vi "Symphony Format Area.vi"(4 "Y Start":i32=255 min=1 max=255 step=1, 5 "Y End":i32=256 min=1 max=256 step=1, 6 "ImageMode":bool, 7 "error in (no error)":errorcluster, 8 "X Start":i32=1023 min=1 max=1023 step=1, 9 "X End":i32=1024 min=1 max=1024 step=1, 10 "numAreas":i32=1) -> (0 "error out":errorcluster, 2 "areas :":i32[][](array[numeric])=[[1], [1], [1], [1024], [256], [1], [256]], 3 "X Size Out":i32=1023 min=1 max=1023 step=1)   [LabVIEW 2019]
panel:
  # "Area#"
  # "X Origin"
  # "Y Origin"
  # "X Size"
  # "Y Size"
  # "X Bin"
  # "Y Bin"
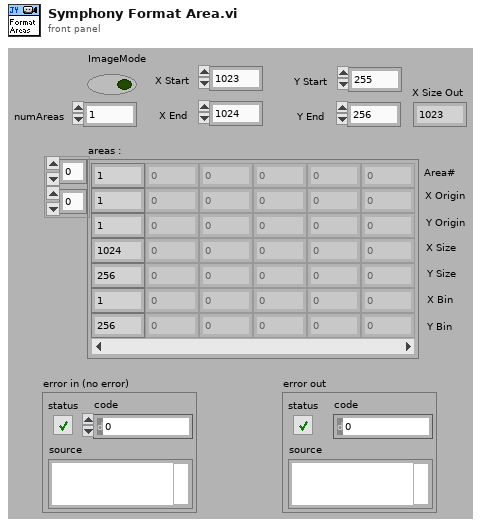
[diagram p1: front panel]
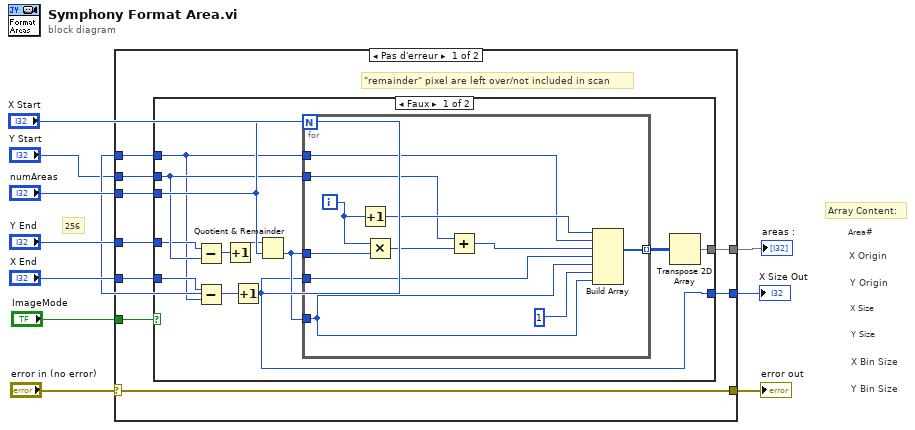
[diagram p0: block diagram]
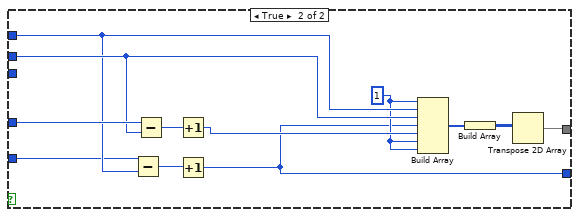
[diagram p2: hidden frame]
diagram:
  # "256"
  # "Array Content:"
  # "Y Bin Size"
  # "X Bin Size"
  # "Y Size"
  # "X Size"
  # "Y Origin"
  # "X Origin"
  # "Area#"
  n1 = case shown="Pas d'erreur" "error in (no error)" {
    selector: "error in (no error)" -> [w17 w55]
    tunnel: "numAreas" -> [w19 _]
    tunnel: [w18 _] -> w9
    tunnel: "X End" -> [w14 _]
    tunnel: "Y End" -> [w15 _]
    tunnel: [w17 w55] -> w5
    tunnel: "X Start" -> [w13 _]
    tunnel: "Y Start" -> [w16 _]
    tunnel: "ImageMode" -> [w12 _]
    tunnel: [w11 _] -> w1
    frame No Error {
      # "\"remainder\" pixel are left over/not included in scan"
      n2 = case shown="Faux" w12 {
        tunnel: w19 -> [w31 _]
        tunnel: [w29 w44] -> w18
        tunnel: w16 -> [w27 w51]
        tunnel: w15 -> [w26 w53]
        tunnel: w14 -> [w24 w47]
        tunnel: w13 -> [w23 w48]
        tunnel: [w20 w43] -> w11
        frame False {
          n3 = Subtract(x=w26, y=w27) -> (x-y=w22:i32)
          n4 = Subtract(x=w24, y=w23) -> (x-y=w21:i32)
          n5 = Increment(x=w22) -> (x+1=w25:i32)
          n6 = Increment(x=w21) -> (x+1=w20:i32)
          n7 = Quotient & Remainder(x=w25, y=w31) -> (floor(x/y)=w28:i32)  [unwired: 1 out]
          n8 = for {
            N: w31 -> [_]
            tunnel: w28 -> [w40]
            tunnel: [w42] -> w30 mode=indexing
            tunnel: w28 -> [w37]
            tunnel: w20 -> [w36]
            tunnel: w23 -> [w35]
            tunnel: w27 -> [w33]
            i -> [w39]
            n9 = Increment(x=w39) -> (x+1=w38:i32)
            n10 = Multiply(x=w39, y=w40) -> (x*y=w32:i32)
            n11 = Add(x=w33, y=w32) -> (x+y=w34:i32)
            n12 = Build Array(w38, w35, w34, w36, w37, 1, w37) -> (w42:i32[])
          }
          n13 = Transpose 2D Array(2D array=w30) -> (transposed array=w29:i32[][])
        }
        frame True {
          w46 = 1 ("numAreas")
          n14 = Subtract(x=w47, y=w48) -> (x-y=w49:i32)
          n15 = Subtract(x=w53, y=w51) -> (x-y=w52:i32)
          n16 = Increment(x=w52) -> (x+1=w50:i32)
          n17 = Increment(x=w49) -> (x+1=w43:i32)
          n18 = Build Array(w46, w48, w51, w43, w50, w46, w46) -> (w54:i32[])
          n19 = Build Array(w54) -> (w45:i32[][])
          n20 = Transpose 2D Array(2D array=w45) -> (transposed array=w44:i32[][])
        }
      }
    }
    frame Error {
    }
  }
  "error out" <- w5
  "areas :" <- w9
  "X Size Out" <- w1
